vi "Handler - Check for Data.vi"(8 "error in (no error)":errorcluster, 11 "RT - Analysis Data in":T2 {"Cutoff Frequncies"."HP Passband" min=1.0 step=1.0 format="%#.4f"; "Cutoff Frequncies"."LP Stopband" min=1.0 step=1.0 format="%#.4f"; "Cutoff Frequncies"."HP Stopband" min=1.0 step=1.0 format="%#.4f"; "Cutoff Frequncies"."LP Passband" min=1.0 step=1.0 format="%#.4f"}) -> (0 "error out":errorcluster, 1 "timed out?":bool, 2 "Raw Data out":T1, 3 "RT - Analysis Data out":T2 {"Cutoff Frequncies"."HP Passband" min=1.0 step=1.0 format="%#.4f"; "Cutoff Frequncies"."LP Stopband" min=1.0 step=1.0 format="%#.4f"; "Cutoff Frequncies"."HP Stopband" min=1.0 step=1.0 format="%#.4f"; "Cutoff Frequncies"."LP Passband" min=1.0 step=1.0 format="%#.4f"})   [LabVIEW 2018]
doc: "This VI waits for data to arrive at the first shared variable. When this variable does NOT timeout, data is pulled from all variables. If the variable does timeout, the VI does nothing. When data is pulled, it is analyzed."
uses:
  Top Level/Shared Controls/Acq Data.ctl
  Private Controls/RT-Analysis Data.ctl
  RT - Analysis.lvlib
  Top Level/Shared Controls/All Data Cluster.ctl
  Top Level/Shared Controls/Post-Analysis Data.ctl
  Top Level/Shared Controls/Calculated Data.ctl
  Top Level/Shared Controls/Analyzed Data Sets.ctl
  Top Level/Shared Controls/Parsed Tag Cluster.ctl
  Private Controls/Parsed Data Arrays.ctl
  Modules/Testing UI 3/Private Controls/Cutoff Frequency.ctl
  Modules/Testing UI 3/Testing UI 3.lvlib
  Top Level/Shared Controls/APU Setup File.ctl
panel:
  out "Data Lagged?":bool
  out "Data Lag":dbl
  # "Highpass Cutoff Frequency"
  # "Lowpass Cutoff Frequency"
  # "Highpass Cutoff Frequency"
  # "Lowpass Cutoff Frequency"
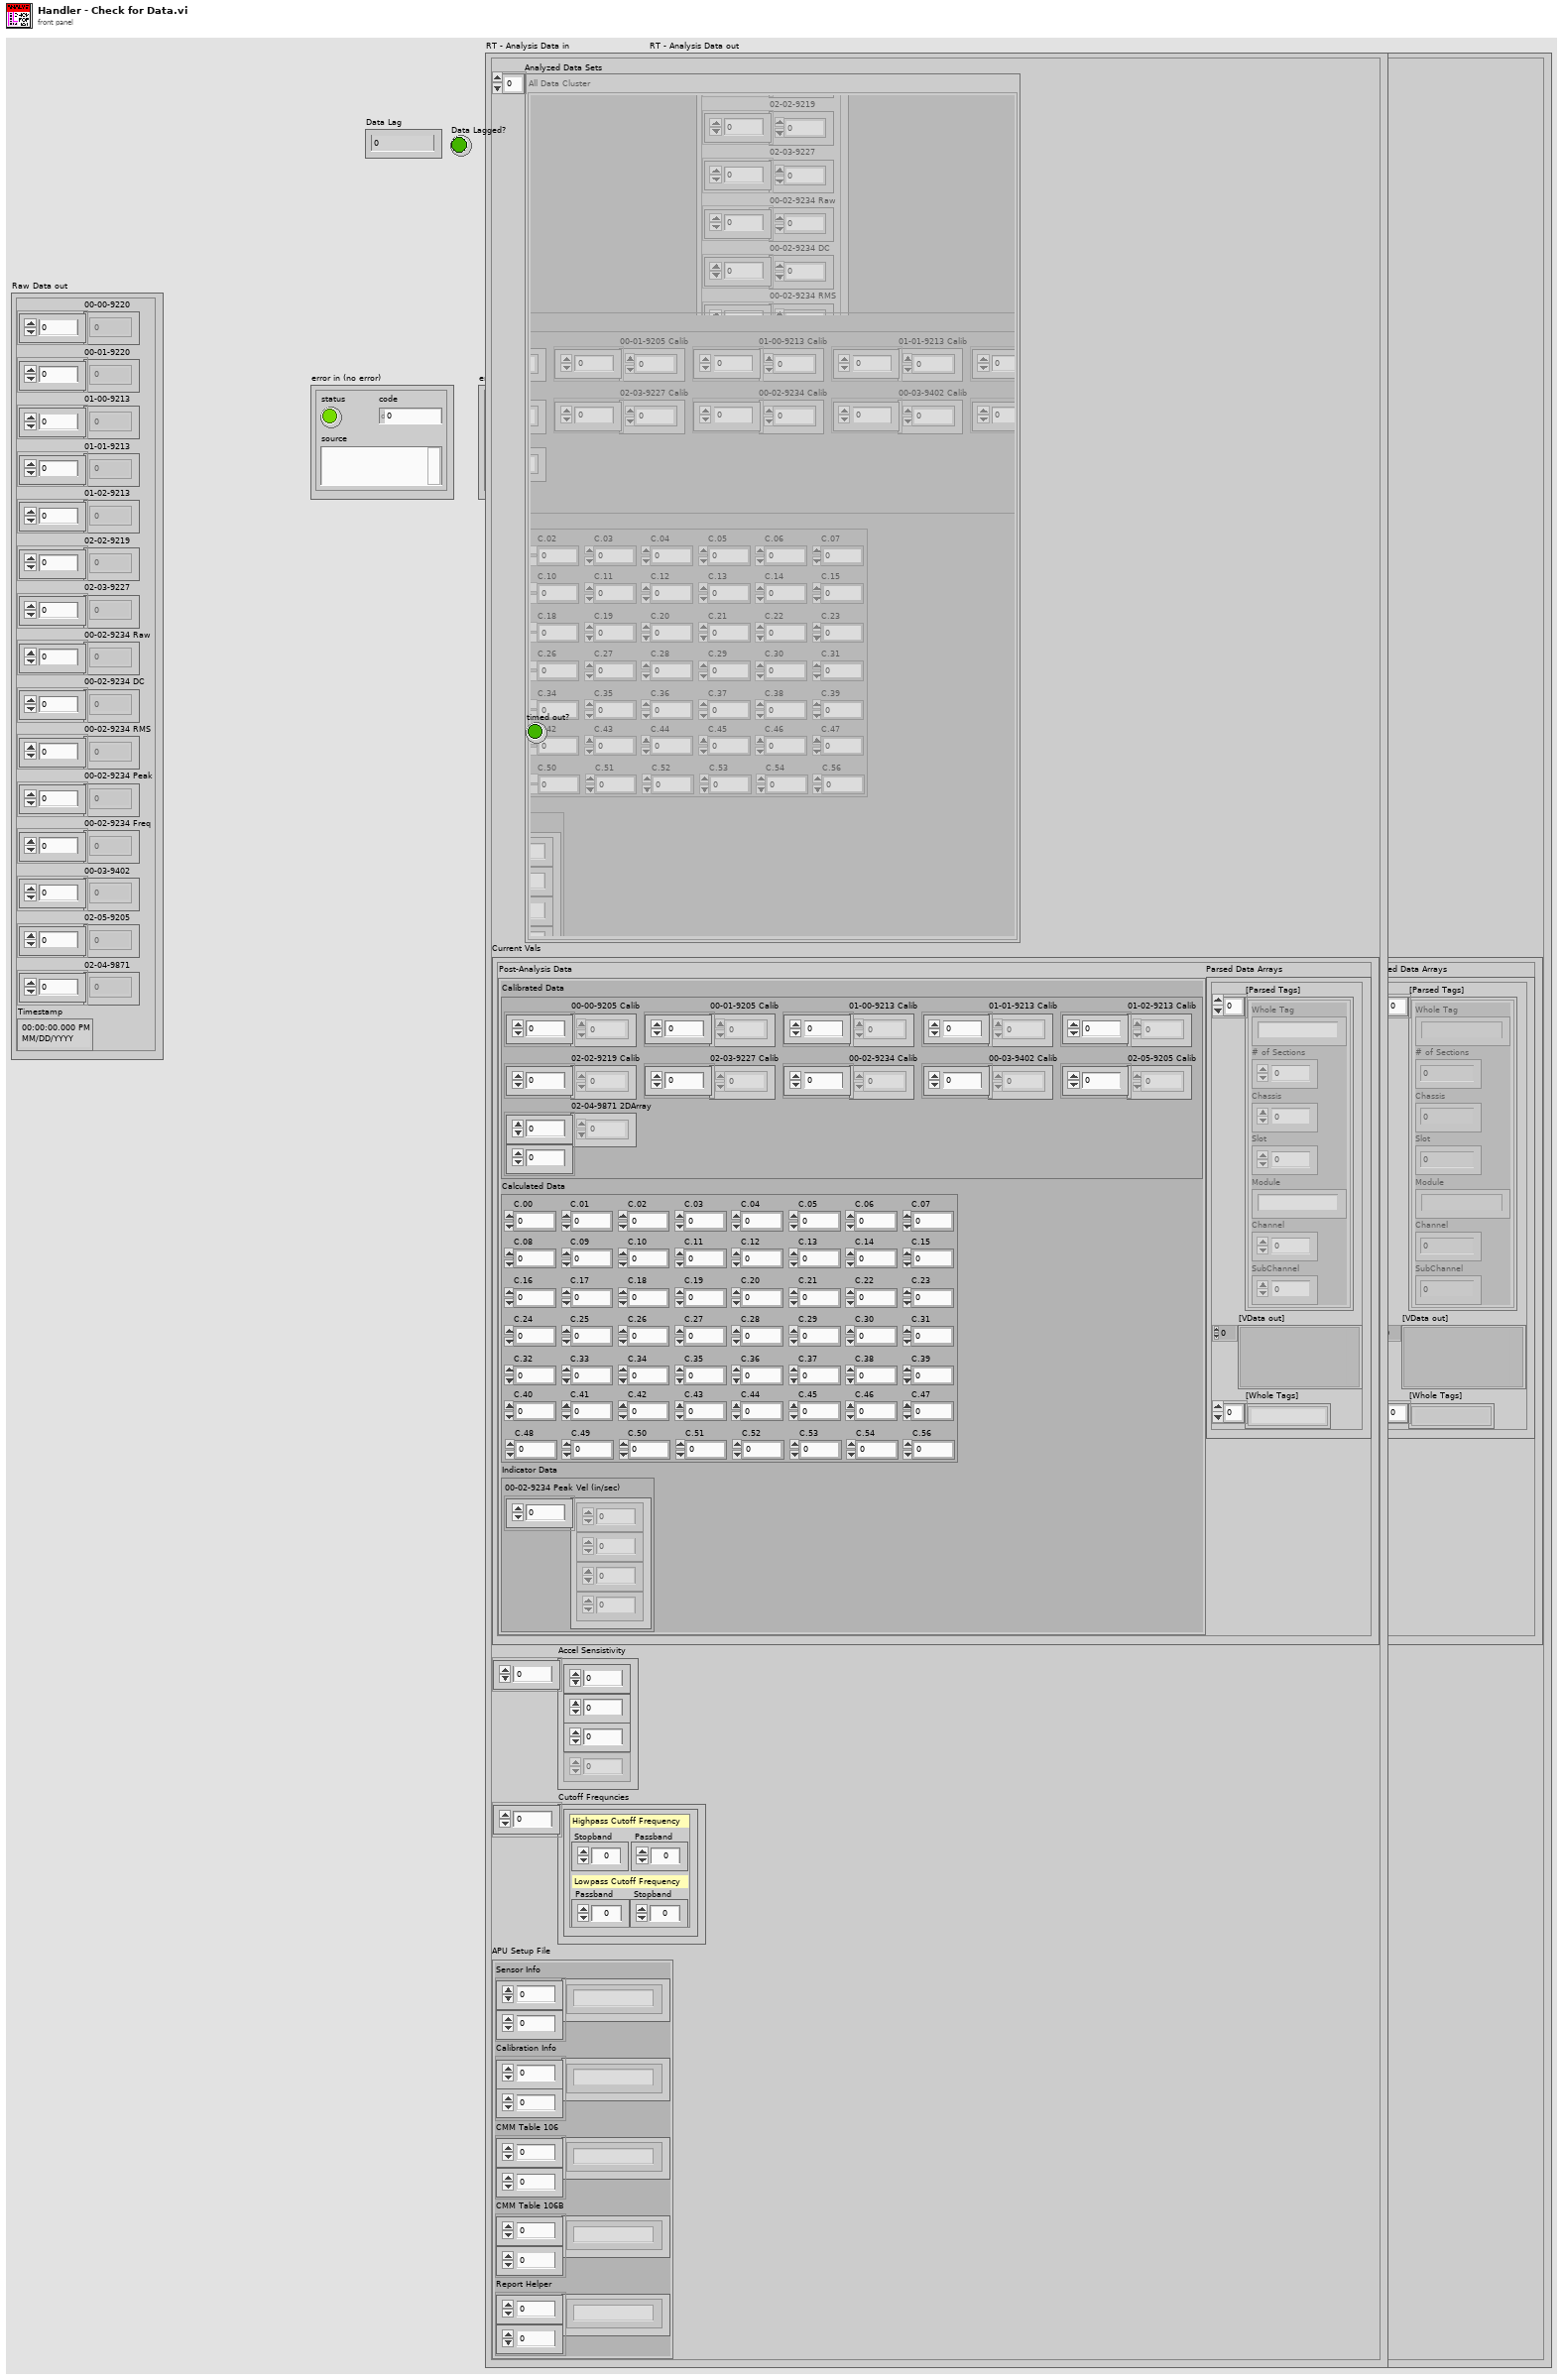
[diagram p1: front panel]
types:
  T1 = typedef "Acq Data.ctl" = cluster{"00-00-9220":dbl[], "00-01-9220":dbl[], "01-00-9213":dbl[], "01-01-9213":dbl[], "01-02-9213":dbl[], "02-02-9219":dbl[], "02-03-9227":dbl[], "00-02-9234 Raw":dbl[], "00-02-9234 DC":dbl[], "00-02-9234 RMS":dbl[], "00-02-9234 Peak":dbl[], "00-02-9234 Freq":dbl[], "00-03-9402":dbl[], "02-05-9205":dbl[], "02-04-9871":dbl[], "Timestamp":timestamp}
  T2 = typedef "RT - Analysis.lvlib/RT-Analysis Data.ctl" = cluster{"Analyzed Data Sets":T3, "Current Vals":cluster{"Post-Analysis Data":T5, "Parsed Data Arrays":T7}, "Accel Sensistivity":dbl[], "Cutoff Frequncies":T9[], "APU Setup File":T10}
  T3 = typedef "Analyzed Data Sets.ctl" = T4[]
  T4 = typedef "All Data Cluster.ctl" = cluster{"Acq Data":T1, "Post-Analysis Data":T5}
  T5 = typedef "Post-Analysis Data.ctl" = cluster{"Calibrated Data":cluster{"00-00-9205 Calib":dbl[], "00-01-9205 Calib":dbl[], "01-00-9213 Calib":dbl[], "01-01-9213 Calib":dbl[], "01-02-9213 Calib":dbl[], "02-02-9219 Calib":dbl[], "02-03-9227 Calib":dbl[], "00-02-9234 Calib":dbl[], "00-03-9402 Calib":dbl[], "02-05-9205 Calib":dbl[], "02-04-9871 2DArray":dbl[][]}, "Calculated Data":T6, "Indicator Data":cluster{"00-02-9234 Peak Vel (in/sec)":dbl[]}}
  T6 = typedef "Calculated Data.ctl" = cluster{"C.00":dbl, "C.01":dbl, "C.02":dbl, "C.03":dbl, "C.04":dbl, "C.05":dbl, "C.06":dbl, "C.07":dbl, "C.08":dbl, "C.09":dbl, "C.10":dbl, "C.11":dbl, "C.12":dbl, "C.13":dbl, "C.14":dbl, "C.15":dbl, "C.16":dbl, "C.17":dbl, "C.18":dbl, "C.19":dbl, "C.20":dbl, "C.21":dbl, "C.22":dbl, "C.23":dbl, "C.24":dbl, "C.25":dbl, "C.26":dbl, "C.27":dbl, "C.28":dbl, "C.29":dbl, "C.30":dbl, "C.31":dbl, "C.32":dbl, "C.33":dbl, "C.34":dbl, "C.35":dbl, "C.36":dbl, "C.37":dbl, "C.38":dbl, "C.39":dbl, "C.40":dbl, "C.41":dbl, "C.42":dbl, "C.43":dbl, "C.44":dbl, "C.45":dbl, "C.46":dbl, "C.47":dbl, "C.48":dbl, "C.49":dbl, "C.50":dbl, "C.51":dbl, "C.52":dbl, "C.53":dbl, "C.54":dbl, "C.56":dbl}
  T7 = typedef "RT - Analysis.lvlib/Parsed Data Arrays.ctl" = cluster{"[Parsed Tags]":T8[], "[VData out]":variant[], "[Whole Tags]":string[]}
  T8 = typedef "Parsed Tag Cluster.ctl" = cluster{"Whole Tag":string, "# of Sections":u8, "Chassis":u8, "Slot":u8, "Module":string, "Channel":u8, "SubChannel":u8}
  T9 = typedef "Testing UI 3.lvlib/Cutoff Frequency.ctl" = cluster{"LP Passband":dbl, "HP Stopband":dbl, "LP Stopband":dbl, "HP Passband":dbl}
  T10 = typedef "APU Setup File.ctl" = cluster{"Sensor Info":string[][], "Calibration Info":string[][], "CMM Table 106":string[][], "CMM Table 106B ":string[][], "Report Helper":string[][]}
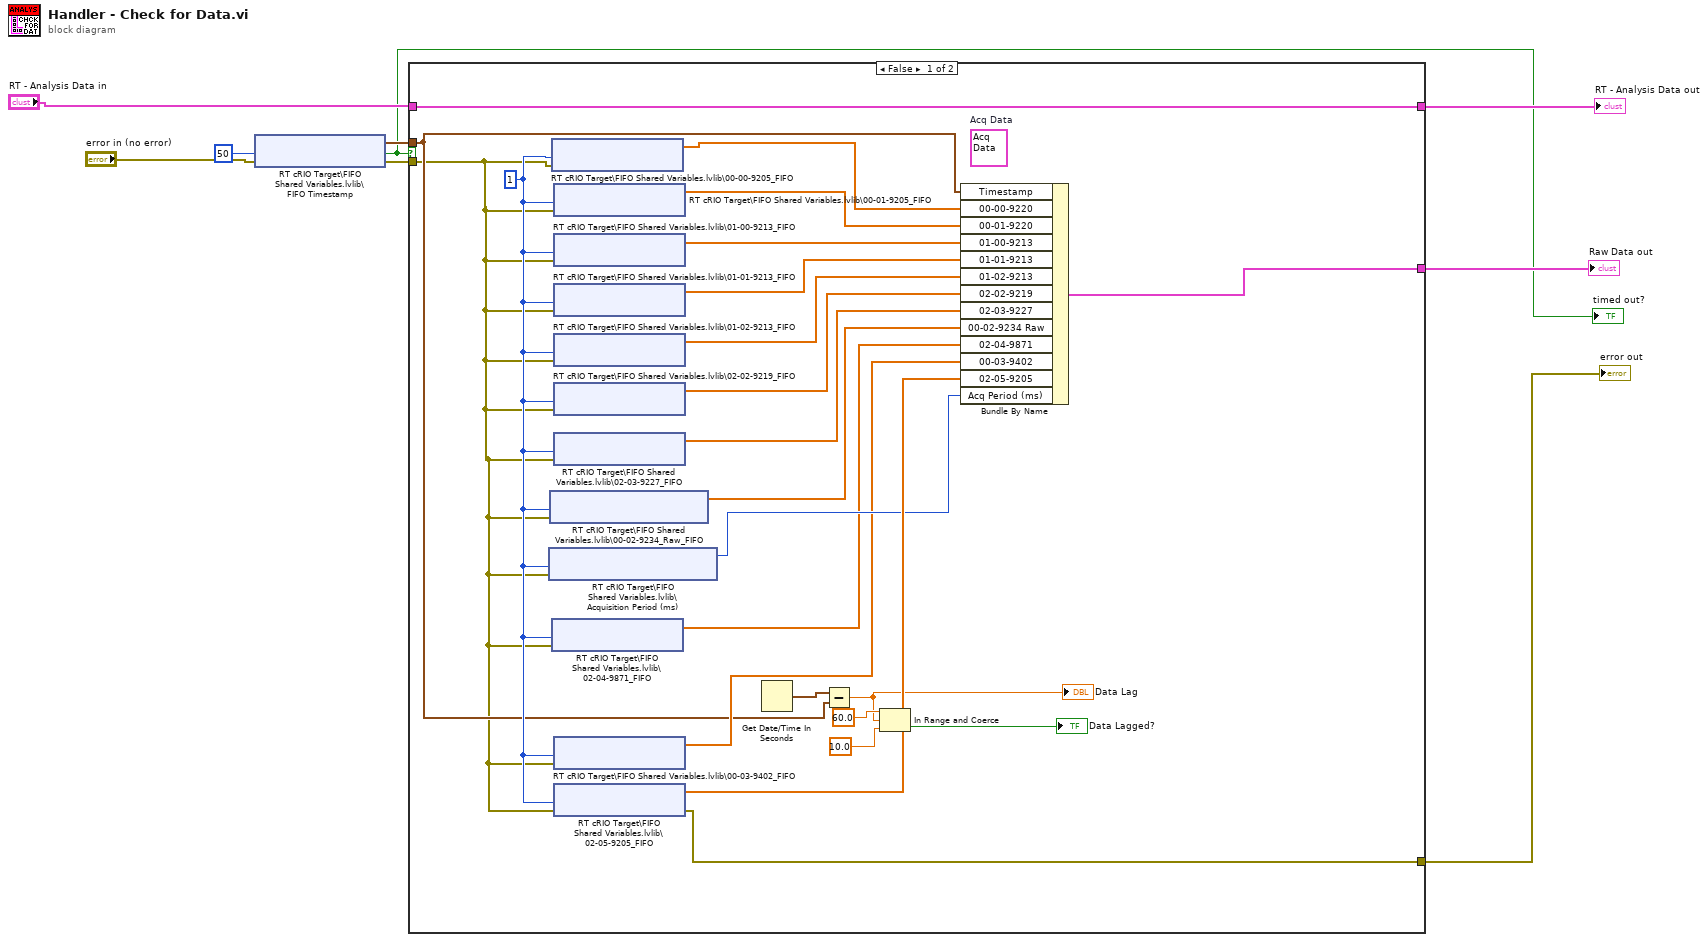
[diagram p0: block diagram]
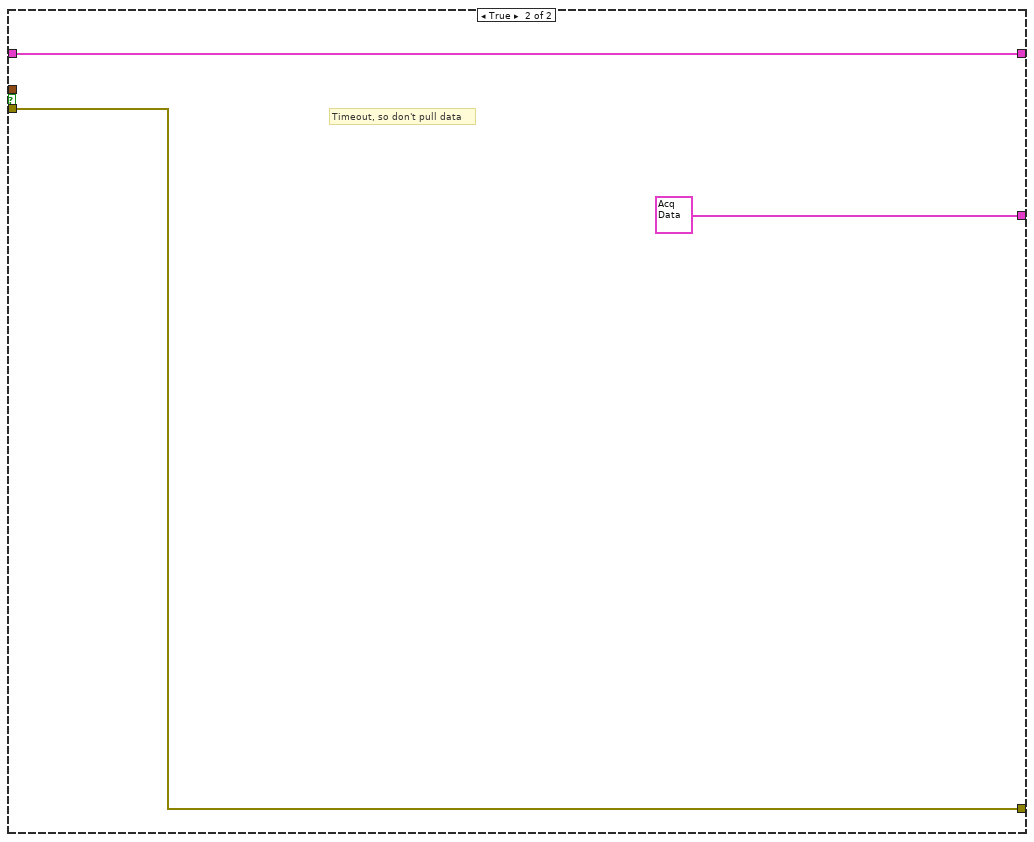
[diagram p2: hidden frame]
diagram:
  n1 = shared-variable "RT cRIO Target\\FIFO Shared Variables.lvlib\\FIFO Timestamp"(error in="error in (no error)", 50 ("ms timeout (0)")) -> (w4:timestamp, error out=w6:errorcluster, w1:bool)
  "timed out?" <- w1
  n2 = case shown="False" w1 {
    tunnel: [w10 T1 {"00-00-9220"=[], "00-01-9220"=[], "01-00-9213"=[], "01-01-9213"=[], "01-02-9213"=[], "02-02-9219"=[], "02-03-9227"=[], "00-02-9234 Raw"=[], "00-02-9234 DC"=[], "00-02-9234 RMS"=[], "00-02-9234 Peak"=[], "00-02-9234 Freq"=[], "00-03-9402"=[], "02-05-9205"=[], "02-04-9871"=[], "Timestamp"=timestamp(0 s since 1904-01-01)} ("Acq Data")] -> w2
    tunnel: w6 -> [w12 w36]
    tunnel: "RT - Analysis Data in" -> [w20 w35]
    tunnel: [w13 w36] -> w3
    tunnel: [w20 w35] -> w9
    tunnel: w4 -> [w14 _]
    frame False {
      (unwired) T1 {"00-00-9220"=[], "00-01-9220"=[], "01-00-9213"=[], "01-01-9213"=[], "01-02-9213"=[], "02-02-9219"=[], "02-03-9227"=[], "00-02-9234 Raw"=[], "00-02-9234 DC"=[], "00-02-9234 RMS"=[], "00-02-9234 Peak"=[], "00-02-9234 Freq"=[], "00-03-9402"=[], "02-05-9205"=[], "02-04-9871"=[], "Timestamp"=timestamp(0 s since 1904-01-01)}  # Acq Data
      w15 = 1 ("ms timeout (0)")
      n3 = shared-variable "RT cRIO Target\\FIFO Shared Variables.lvlib\\Acquisition Period (ms)"(error in=w12, w15) -> (w25:i64)  [unwired: 2 out]
      n4 = shared-variable "RT cRIO Target\\FIFO Shared Variables.lvlib\\00-02-9234_Raw_FIFO"(error in=w12, w15) -> (w26:sgl[])  [unwired: 2 out]
      n5 = shared-variable "RT cRIO Target\\FIFO Shared Variables.lvlib\\00-00-9205_FIFO"(error in=w12, w15) -> (w16:dbl[])  [unwired: 2 out]
      n6 = shared-variable "RT cRIO Target\\FIFO Shared Variables.lvlib\\02-04-9871_FIFO"(error in=w12, w15) -> (w21:dbl[])  [unwired: 2 out]
      n7 = shared-variable "RT cRIO Target\\FIFO Shared Variables.lvlib\\00-01-9205_FIFO"(error in=w12, w15) -> (w33:dbl[])  [unwired: 2 out]
      n8 = shared-variable "RT cRIO Target\\FIFO Shared Variables.lvlib\\01-00-9213_FIFO"(error in=w12, w15) -> (w32:dbl[])  [unwired: 2 out]
      n9 = shared-variable "RT cRIO Target\\FIFO Shared Variables.lvlib\\01-01-9213_FIFO"(error in=w12, w15) -> (w31:dbl[])  [unwired: 2 out]
      n10 = shared-variable "RT cRIO Target\\FIFO Shared Variables.lvlib\\01-02-9213_FIFO"(error in=w12, w15) -> (w30:dbl[])  [unwired: 2 out]
      n11 = shared-variable "RT cRIO Target\\FIFO Shared Variables.lvlib\\02-02-9219_FIFO"(error in=w12, w15) -> (w29:dbl[])  [unwired: 2 out]
      n12 = shared-variable "RT cRIO Target\\FIFO Shared Variables.lvlib\\02-03-9227_FIFO"(error in=w12, w15) -> (w28:dbl[])  [unwired: 2 out]
      n13 = shared-variable "RT cRIO Target\\FIFO Shared Variables.lvlib\\00-03-9402_FIFO"(error in=w12, w15) -> (w22:sgl[])  [unwired: 2 out]
      n14 = shared-variable "RT cRIO Target\\FIFO Shared Variables.lvlib\\02-05-9205_FIFO"(error in=w12, w15) -> (w27:dbl[], error out=w13:errorcluster)  [unwired: 1 out]
      n15 = Get Date/Time In Seconds() -> (seconds since 1Jan1904=w23:timestamp)
      n16 = Subtract(x=w23, y=w14) -> (x-y=w18:dbl)
      "Data Lag" <- w18
      n17 = In Range and Coerce(upper limit=60.0, x=w18, lower limit=10.0 ("y")) -> (In Range?=→"Data Lagged?":bool)  [unwired: 1 out]
      n18 = Bundle By Name("Timestamp"=w14, "00-00-9220"=w16, "00-01-9220"=w33, "01-00-9213"=w32, "01-01-9213"=w31, "01-02-9213"=w30, "02-02-9219"=w29, "02-03-9227"=w28, "00-02-9234 Raw"=w26, "02-04-9871"=w21, "00-03-9402"=w22, "02-05-9205"=w27, "Acq Period (ms)"=w25) -> (w10:cluster{}, w11:cluster{})
    }
    frame True {
      # "Timeout, so don't pull data"
    }
  }
  "RT - Analysis Data out" <- w9
  "error out" <- w3
  "Raw Data out" <- w2
